vi "trigonometrik_kullanıldı.vi"() -> ()   [LabVIEW 2019]
panel:
  in  "Açý":string
  out "Sonuç":dbl
  in  "Trig. Ýþlem Türü":string
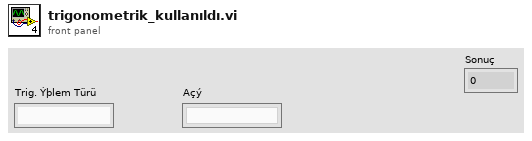
[diagram p1: front panel]
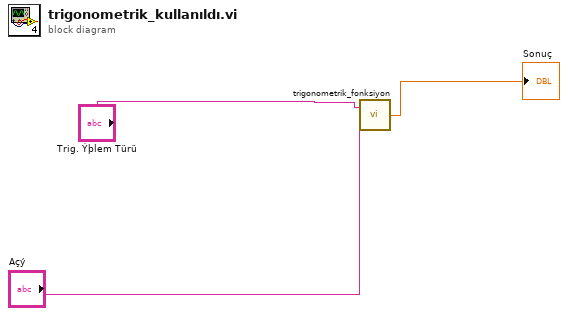
[diagram p0: block diagram]
diagram:
  n1 = call "trigonometrik_fonksiyon.vi"("Açý"="Açý", "Trigonometrik Ýþlem Türü"="Trig. Ýþlem Türü") -> ("Sonuç"=→"Sonuç":dbl)
